vi "Read Secondary Status Byte.vi"(7 "Read Secondary Status Bit? (F)":bool, 8 "error in (no error)":errorcluster, 9 "Secondary Status Bit (Triggered)":T1, 11 "VISA resource name":refnum<visa-resource-name>) -> (0 "error out":errorcluster, 1 "Secondary Status Bit":u8, 2 "Secondary Status Byte":bool[](array[boolean]), 3 "VISA resource name out":refnum<visa-resource-name>)   [LabVIEW 2013, in "SRS SR400.lvlib"]
doc: "<B>SI { j }</B>\n\nThe SI command reads the secondary status byte. (See the following section for a definition of the secondary status byte). j designates one bit, 0-2, of the byte. If j is included, the designated bit of the secondary status byte is returned (\"0\" or \"1\"). The bit which is read is then reset. If j is absent, the value of the entire byte is returned (0-7) and all secondary status bits are then reset.\n\nThe definitions for each bit of the secondary status byte are given below:\n\n<B>Bit 0</B>\nTriggered. This bit is set when the gate generator is triggered.\n\n<B>Bit 1</B>\nInhibited. This bit is set when the discriminators are inhibited.\n\n<B>Bit 2</B>\nCounting. This bit samples the state of the counters. If counting is in progress when this bit is polled, a 1 is returned, otherwise a 0 is returned."
uses:
  <instrlib>/SRS SR400/SRS SR400.lvlib
  <instrlib>/SRS SR400/Public/Typedefs/Secondary Status Bit.ctl
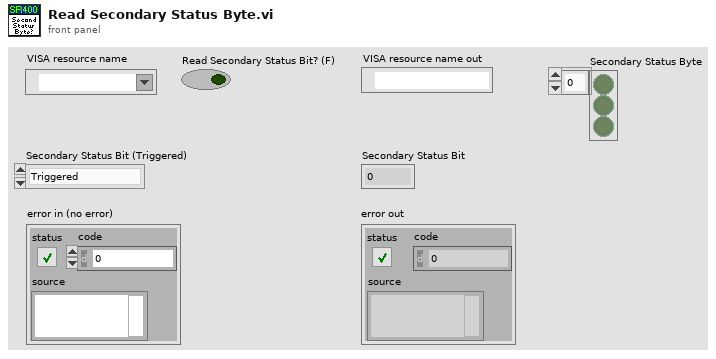
[diagram p1: front panel]
types:
  T1 = typedef "SRS SR400.lvlib/Secondary Status Bit.ctl" = enum16{"Triggered", "Inhibited", "Counting"}
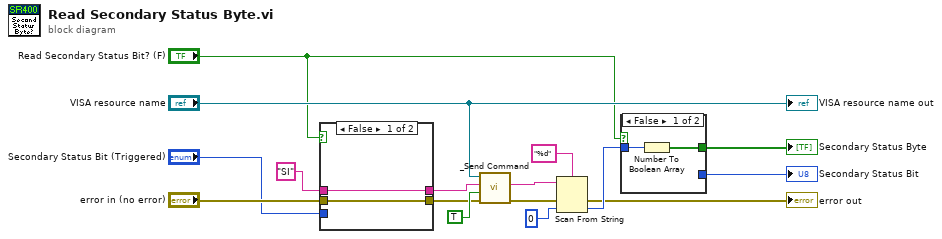
[diagram p0: block diagram]
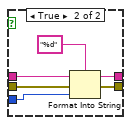
[diagram p3: hidden frame]
diagram:
  n1 = case shown="False" "Read Secondary Status Bit? (F)" {
    tunnel: "error in (no error)" -> [w17 w24]
    tunnel: [w17 w23] -> w6
    tunnel: "SI" ("Command") -> [w18 w21]
    tunnel: "Secondary Status Bit (Triggered)" -> [_ w20]
    tunnel: [w18 w19] -> w3
    frame False {
    }
    frame True {
      n2 = Format Into String(format string="%d", initial string=w21, error in=w24, w20) -> (resulting string=w19:string, error out=w23:errorcluster)
    }
  }
  n3 = call <instrlib>:"_Send Command.vi"("error in (no error)"=w6, "Read Value? (F)"=TRUE ("Query? (F)"), "Command"=w3, "VISA resource name"="VISA resource name") -> ("error out"=w10:errorcluster, "Response"=w11:string)  [unwired: 5 in, 1 out]
  n4 = Scan From String(format string="%d", input string=w11, error in=w10, default 1=u8 0 ("default value 1")) -> (error out=→"error out":errorcluster, output 1=w12:u8)  [unwired: 1 in, 2 out]
  n5 = case shown="False" "Read Secondary Status Bit? (F)" {
    tunnel: [w26 _] -> w15
    tunnel: w12 -> [w25 w27]
    tunnel: [_ w27] -> w1
    frame False {
      n6 = Number To Boolean Array(number=w25) -> (Boolean array=w26:bool[])
    }
    frame True {
    }
  }
  "Secondary Status Byte" <- w15
  "Secondary Status Bit" <- w1
  "VISA resource name out" <- "VISA resource name"
